vi "FPGA_PPG_read_file.vi"(0 "file_in":path, 5 "error in (no error)":errorcluster) -> (14 "file_out":path, 16 "linesWithError":cluster{"Zeile":i32, "Code":i32}[](array[cluster]), 17 "cmd_lines":string[](array[string]), 18 "cmd_number":i32, 19 "error out":errorcluster)   [LabVIEW 2014, in "NI-FPGA_PPG_Driver.lvlib"]
doc: "Reads commands to be written to the FPGA from a file."
uses:
  NI-FPGA_PPG_Driver.lvlib
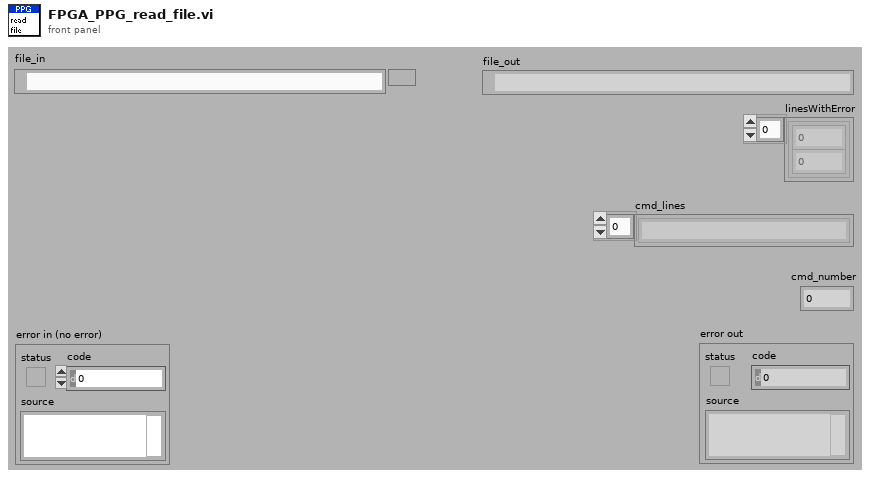
[diagram p1: front panel]
types:
  T1 = enum16{"open", "replace", "create", "open or create", "replace or create", "replace or create with confirmation"}
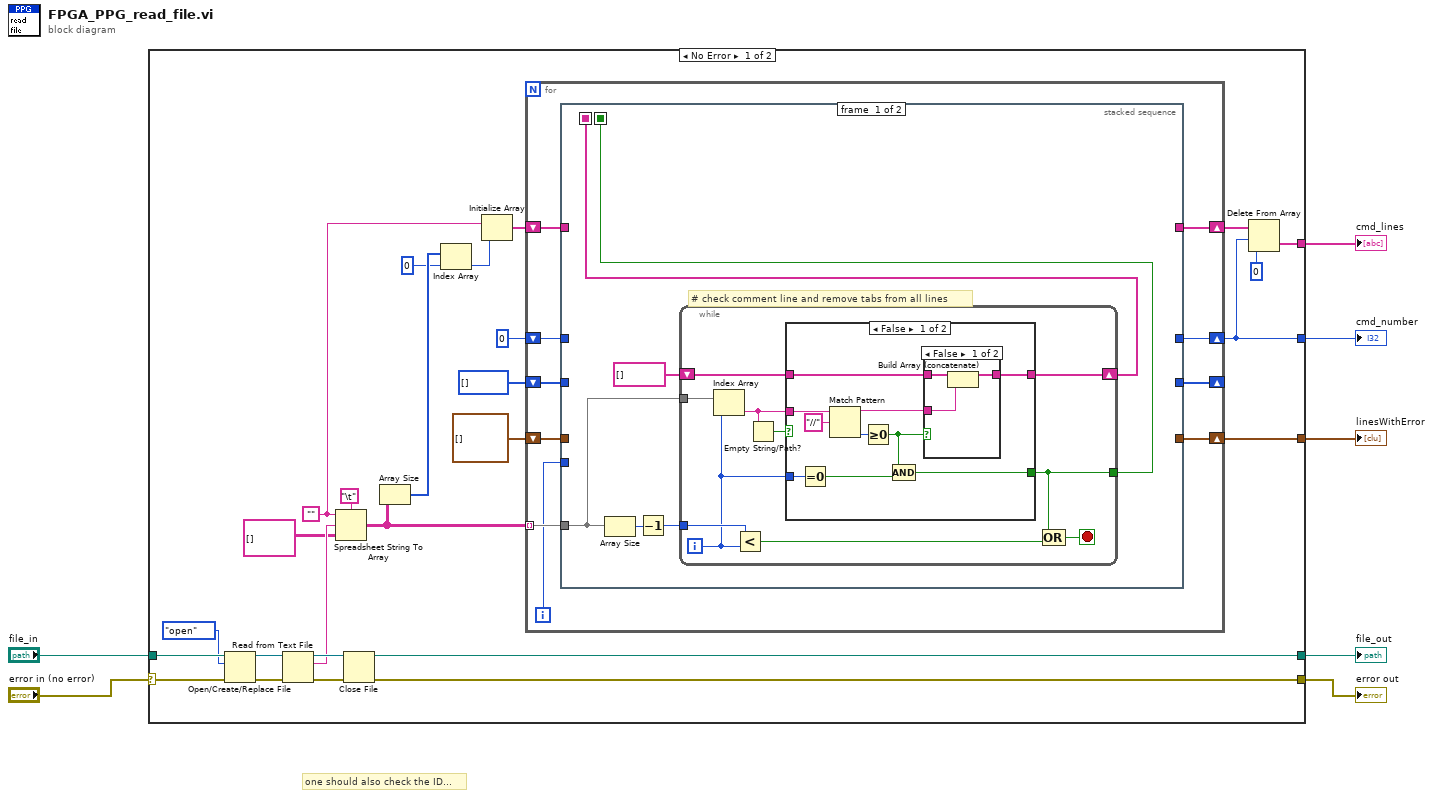
[diagram p0: block diagram]
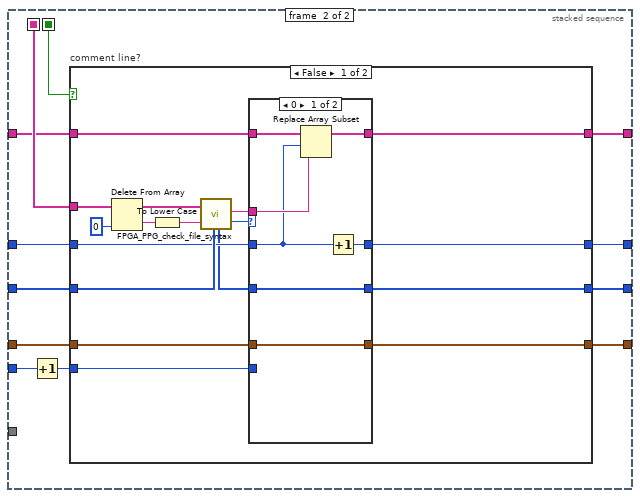
[diagram p4: hidden frame]
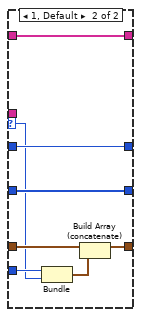
[diagram p5: hidden frame]
diagram:
  # "one should also check the ID..."
  n1 = case shown="No Error" "error in (no error)" {
    selector: "error in (no error)" -> [w33 w124]
    tunnel: [w31 w124] -> w6
    tunnel: "file_in" -> [w32 w123]
    tunnel: [w30 w123] -> w4
    tunnel: [w10 _] -> w2
    tunnel: [w18 _] -> w3
    tunnel: [w8 _] -> w1
    frame No Error {
      w16 = "" ("format string")
      n2 = Open/Create/Replace File(file path (use dialog)=w32, error in=w33, operation (0:open)=T1."open") -> (refnum out=w27:refnum<file>, error out=w28:errorcluster)  [unwired: 3 in, 1 out]
      n3 = Read from Text File(file (use dialog)=w27, error in=w28) -> (refnum out=w25:refnum<file>, text=w24:string, error out=w26:errorcluster)  [unwired: 2 in, 1 out]
      n4 = Spreadsheet String To Array(delimiter (Tab)="\t", format string=w16, spreadsheet string=w24, array type (2D Dbl)=string[][] []) -> (array=w17:string[][])
      n5 = Close File(refnum=w25, error in=w26) -> (path=w30:path, error out=w31:errorcluster)
      n6 = Array Size(array=w17) -> (size(s)=w15:i32[])
      n7 = Index Array(array=w15, index=0) -> (element=w14:i32)
      n8 = Initialize Array(w16, w14) -> (w13:string[])
      n9 = for {
        tunnel: w17 -> [w43] mode=indexing
        shift-right: [w41] -> _
        shift-left: u32[] [] -> [w42]
        shift-right: [w39] -> w10
        shift-left: 0 -> [w40]
        shift-right: [w36] -> w18
        shift-left: cluster{i32, i32}[] [] -> [w38]
        shift-right: [w35] -> w11
        shift-left: w13 -> [w34]
        i -> [w37]
        n10 = stacked-sequence {
          seq-local: [w44 _] -> [_ w85]
          seq-local: [w45 _] -> [_ w86]
          tunnel: w43 -> [w48 _]
          tunnel: w42 -> [_ w84]
          tunnel: [_ w83] -> w41
          tunnel: w40 -> [_ w82]
          tunnel: [_ w81] -> w39
          tunnel: w38 -> [_ w80]
          tunnel: w37 -> [_ w76]
          tunnel: [_ w79] -> w36
          tunnel: [_ w78] -> w35
          tunnel: w34 -> [_ w77]
          frame #0 {
            # "# check comment line and remove tabs from all lines"
            n11 = Array Size(array=w48) -> (size(s)=w47:i32)
            n12 = Decrement(x=w47) -> (x-1=w46:i32)
            n13 = while {
              shift-right: [w58] -> w44
              shift-left: string[] [] -> [w59]
              tunnel: w48 -> [w56]
              tunnel: w46 -> [w54]
              tunnel: [w50] -> w45
              i -> [w53]
              stop <- w51 stop-if-true
              n14 = Index Array(array=w56, index=w53) -> (element=w55:string)
              n15 = Less?(x=w54, y=w53) -> (x < y?=w52:bool)
              n16 = Empty String/Path?(string/path=w55) -> (empty?=w57:bool)
              n17 = case shown="False" w57 {
                tunnel: w59 -> [w69 w74]
                tunnel: [w68 w74] -> w58
                tunnel: w55 -> [w67 _]
                tunnel: w53 -> [w63 _]
                tunnel: [w60 _] -> w50
                frame False {
                  n18 = Equal To 0?(x=w63) -> (x = 0?=w62:bool)
                  n19 = Match Pattern(string=w67, regular expression="//") -> (before substring=w65:string, offset past match=w64:i32)  [unwired: 1 in, 2 out]
                  n20 = Greater Or Equal To 0?(x=w64) -> (x >= 0?=w61:bool)
                  n21 = Compound Arithmetic op=AND(w61, w62) -> (w60:bool)
                  n22 = case shown="False" w61 {
                    tunnel: w69 -> [w72 w73]
                    tunnel: [w71 w73] -> w68
                    tunnel: w65 -> [w70 _]
                    frame False {
                      n23 = Build Array (concatenate)(w72, w70) -> (w71:string[])
                    }
                    frame True {
                    }
                  }
                }
                frame True {
                }
              }
              n24 = Compound Arithmetic op=OR(w50, w52) -> (w51:bool)
            }
          }
          frame #1 {
            n25 = Increment(x=w76) -> (x+1=w75:i32)
            n26 = case "comment line?" shown="False" w86 {
              tunnel: w85 -> [w103 _]
              tunnel: w84 -> [w98 w122]
              tunnel: [w93 w122] -> w83
              tunnel: w82 -> [w97 w121]
              tunnel: [w96 w121] -> w81
              tunnel: w80 -> [w92 w120]
              tunnel: w75 -> [w91 _]
              tunnel: [w90 w120] -> w79
              tunnel: [w88 w119] -> w78
              tunnel: w77 -> [w87 w119]
              frame False {
                n27 = Delete From Array(array=w103, index=0) -> (deleted portion=w101:string, array with subset deleted=w100:string[])  [unwired: 1 in]
                n28 = To Lower Case(string=w101) -> (all lower case string=w99:string)
                n29 = call "FPGA_PPG_check_file_syntax.vi"("cmd_data"=w100, "cmd"=w99, "jump_data_tmp_in"=w98) -> ("jump_data_tmp_out"=w95:u32[], "cmd_line"=w89:string, "codeOfError"=w94:i32)  [unwired: 14 in]
                n30 = case shown="0" w94 {
                  selector: w94 -> [_ w113]
                  tunnel: w97 -> [w104 w118]
                  tunnel: [w110 w118] -> w96
                  tunnel: w95 -> [w109 w117]
                  tunnel: [w109 w117] -> w93
                  tunnel: w92 -> [w108 w116]
                  tunnel: w91 -> [_ w114]
                  tunnel: [w108 w115] -> w90
                  tunnel: w89 -> [w105 _]
                  tunnel: [w107 w111] -> w88
                  tunnel: w87 -> [w106 w111]
                  frame 0 {
                    n31 = Replace Array Subset(array=w106, new element=w105, index=w104) -> (w107:string[])
                    n32 = Increment(x=w104) -> (x+1=w110:i32)
                  }
                  frame 1, Default {
                    n33 = Bundle(w114, w113) -> (w112:cluster{i32, i32})  [unwired: 1 in]
                    n34 = Build Array (concatenate)(w116, w112) -> (w115:cluster{i32, i32}[])
                  }
                }
              }
              frame True {
              }
            }
          }
        }
      }
      n35 = Delete From Array(array=w11, length=w10, index=0) -> (deleted portion=w8:string[])  [unwired: 1 out]
    }
    frame Error {
    }
  }
  "error out" <- w6
  "file_out" <- w4
  "linesWithError" <- w3
  "cmd_number" <- w2
  "cmd_lines" <- w1
